vi "GPS.vi"() -> (0 "GPS error out":errorcluster caption="error out")   [LabVIEW 2016]
uses:
  DLL/Checksum_(T_F).dll
panel:
  in  "stop?":bool
  in  "GPS error in":errorcluster
  in  "GPS Baud rate":u32(ring)=38400 items=["Auto Connect"=0, "300"=300, "600"=600, "1200"=1200, "2400"=2400, "4800"=4800, "9600"=9600, "19200"=19200, "38400"=38400, "57600"=57600, "115200"=115200]
  out "GPS port out":refnum<visa-resource-name>
  out "Time":string
  out "N/S":string
  out "E/W":string
  out "Chechsum 부분":string
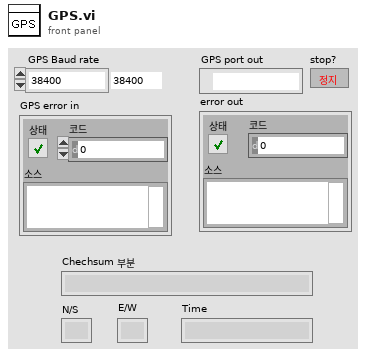
[diagram p1: front panel]
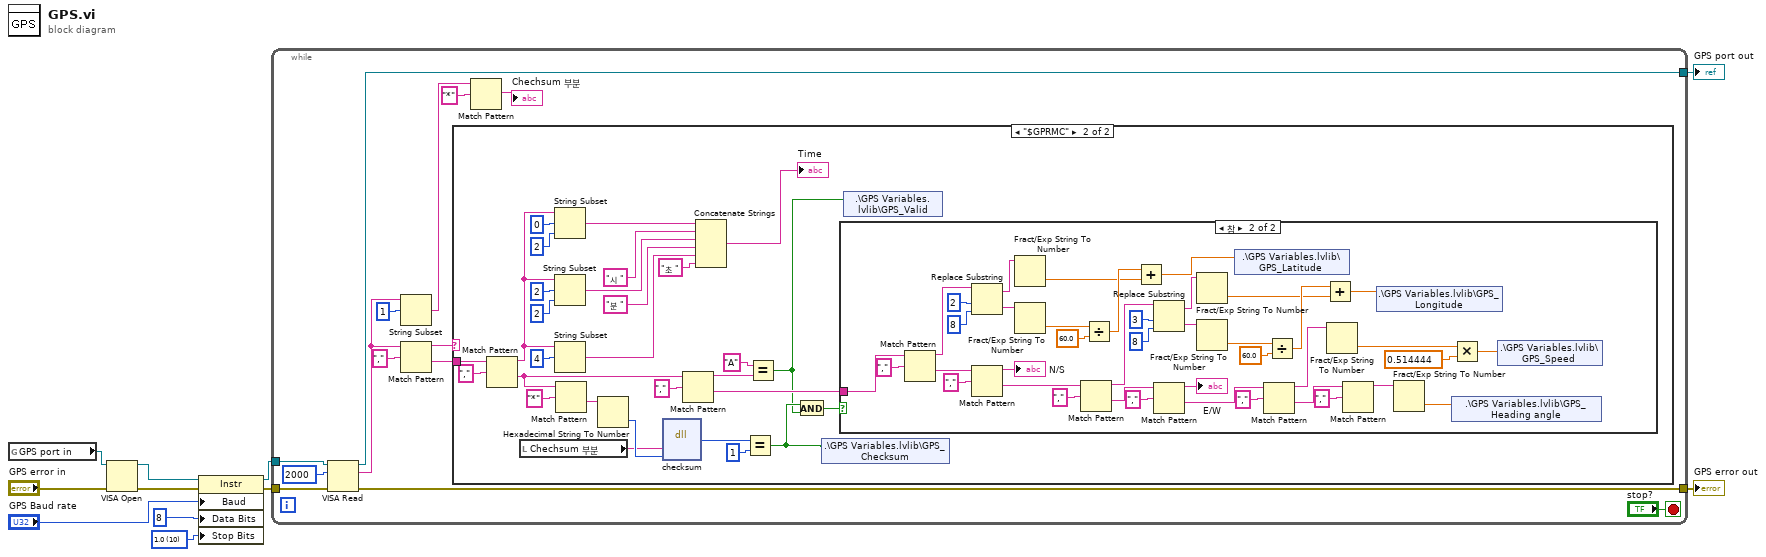
[diagram p0: block diagram]
diagram:
  w8 = u16 10 items=["1.0"=10, "1.5"=15, "2.0"=20] ("Serial Settings:Stop Bits")
  n1 = global read "[GV]_GPS Port NUM.vi" "GPS port in"() -> (w1:refnum<visa-resource-name>)
  n2 = VISA Open(error in (no error)="GPS error in", VISA resource name=w1) -> (VISA resource name=w2:refnum<visa-resource-name>, error out=w6:errorcluster)  [unwired: 3 in]
  n3 = property class="Instr"(reference=w2, error in=w6, "Baud"="GPS Baud rate", "Data Bits"=u16 8 ("Serial Settings:Data Bits"), "Stop Bits"=w8) -> (reference out=w4:refnum<visa-resource-name>, error out=w3:errorcluster)
  n4 = while {
    tunnel: w4 -> [w17]
    tunnel: w3 -> [w16]
    tunnel: [w14] -> w10
    tunnel: [w13] -> w11
    stop <- "stop?" stop-if-true
    n5 = VISA Read(VISA resource name=w17, byte count=u32 2000 ("바이트 카운트"), error in (no error)=w16) -> (VISA resource name out=w14:refnum<visa-resource-name>, read buffer=w18:string, error out=w13:errorcluster)  [unwired: 1 out]
    n6 = String Subset(string=w18, offset (0)=1 ("오프셋(0)")) -> (substring=w19:string)  [unwired: 1 in]
    n7 = Match Pattern(string=w18, regular expression="," ("정규식")) -> (before substring=w24:string, after substring=w23:string)  [unwired: 1 in, 2 out]
    n8 = case shown="\"$GPRMC\"" w24 {
      tunnel: w23 -> [_ w53]
      frame "거짓", Default {
      }
      frame "$GPRMC" {
        n9 = Match Pattern(string=w53, regular expression="," ("정규식")) -> (before substring=w38:string, after substring=w35:string)  [unwired: 1 in, 2 out]
        n10 = local read "Chechsum 부분"() -> (w28:string)
        n11 = String Subset(string=w38, offset (0)=0 ("오프셋(0)"), length (rest)=2 ("길이(나머지)")) -> (substring=w44:string)
        n12 = String Subset(string=w38, offset (0)=2 ("오프셋(0)"), length (rest)=2 ("길이(나머지)")) -> (substring=w47:string)
        n13 = String Subset(string=w38, offset (0)=4 ("오프셋(0)")) -> (substring=w50:string)  [unwired: 1 in]
        n14 = Match Pattern(string=w35, regular expression="*" ("정규식")) -> (after substring=w31:string)  [unwired: 1 in, 3 out]
        n15 = Hexadecimal String To Number(string=w31) -> (number=w34:u32)  [unwired: 2 in, 1 out]
        n16 = dll-call lib="PTH2abs CUsersuserDesktop[Github]_GPS Teamlabview_program(ììì¤ì¸ ëª¨ë  Vi, dllíì¼ ëª¨ìì ì²´íë¡ê·¸ë¨DLLChecksum_(T_F).dll" fn="checksum"("NMEA string"=w28, "Checksum"=w34) -> ("반환 타입"=w33:i16)  [unwired: 5 in, 2 out]
        n17 = Match Pattern(string=w35, regular expression="," ("정규식")) -> (before substring=w37:string, after substring=w29:string)  [unwired: 1 in, 2 out]
        n18 = Concatenate Strings(w44, "시 ", w47, "분 ", w50, "초 ") -> (→"Time":string)
        n19 = Equal?(x=w33, y=i16 1) -> (x = y?=w27:bool)
        n20 = Equal?(x="A" ("y"), y=w37) -> (x = y?=w26:bool)
        n21 = And(x=w27, y=w26) -> (x .and. y?=w30:bool)
        n22 = shared-variable ".\\GPS Variables.lvlib\\GPS_Checksum"(w27) -> ()  [unwired: 1 in, 1 out]
        n23 = case shown="참" w30 {
          tunnel: w29 -> [_ w94]
          frame False {
          }
          frame True {
            n24 = Match Pattern(string=w94, regular expression="," ("정규식")) -> (before substring=w76:string, after substring=w75:string)  [unwired: 1 in, 2 out]
            n25 = Replace Substring(2:8 ("위도_길이(부분 문자열의 길이)"), 3:2 ("위도_오프셋"), 5:w76) -> (0:w88:string, 1:w87:string)  [unwired: 1 in]
            n26 = Match Pattern(string=w75, regular expression="," ("정규식")) -> (before substring=→"N/S":string, after substring=w72:string)  [unwired: 1 in, 2 out]
            n27 = Fract/Exp String To Number(string=w87) -> (number=w85:dbl)  [unwired: 1 in, 3 out]
            n28 = Fract/Exp String To Number(string=w88) -> (number=w89:dbl)  [unwired: 1 in, 3 out]
            n29 = Match Pattern(string=w72, regular expression="," ("정규식")) -> (before substring=w71:string, after substring=w68:string)  [unwired: 1 in, 2 out]
            n30 = Divide(x=w89, y=60.0) -> (x/y=w86:dbl)
            n31 = Add(x=w86, y=w85) -> (x+y=w57:dbl)
            n32 = Replace Substring(2:8 ("경도_길이(부분 문자열의 길이)"), 3:3 ("경도_오프셋(0)"), 5:w71) -> (0:w81:string, 1:w80:string)  [unwired: 1 in]
            n33 = Match Pattern(string=w68, regular expression="," ("정규식")) -> (before substring=→"E/W":string, after substring=w65:string)  [unwired: 1 in, 2 out]
            n34 = Fract/Exp String To Number(string=w80) -> (number=w78:dbl)  [unwired: 4 out]
            n35 = Fract/Exp String To Number(string=w81) -> (number=w70:dbl)  [unwired: 4 out]
            n36 = shared-variable ".\\GPS Variables.lvlib\\GPS_Latitude"(w57) -> ()  [unwired: 1 in, 1 out]
            n37 = Match Pattern(string=w65, regular expression="," ("정규식")) -> (before substring=w62:string, after substring=w60:string)  [unwired: 1 in, 2 out]
            n38 = Divide(x=w70, y=60.0) -> (x/y=w79:dbl)
            n39 = Add(x=w79, y=w78) -> (x+y=w56:dbl)
            n40 = Fract/Exp String To Number(string=w62) -> (number=w63:dbl)  [unwired: 3 in, 1 out]
            n41 = Match Pattern(string=w60, regular expression="," ("정규식")) -> (before substring=w59:string)  [unwired: 1 in, 3 out]
            n42 = shared-variable ".\\GPS Variables.lvlib\\GPS_Longitude"(w56) -> ()  [unwired: 1 in, 1 out]
            n43 = Fract/Exp String To Number(string=w59) -> (number=w58:dbl)  [unwired: 3 in, 1 out]
            n44 = Multiply(x=w63, y=0.514444) -> (x*y=w55:dbl)
            n45 = shared-variable ".\\GPS Variables.lvlib\\GPS_Heading angle"(w58) -> ()  [unwired: 1 in, 1 out]
            n46 = shared-variable ".\\GPS Variables.lvlib\\GPS_Speed"(w55) -> ()  [unwired: 1 in, 1 out]
          }
        }
        n47 = shared-variable ".\\GPS Variables.lvlib\\GPS_Valid"(w26) -> ()  [unwired: 1 in, 1 out]
      }
    }
    n48 = Match Pattern(string=w19, regular expression="*" ("정규식")) -> (before substring=→"Chechsum 부분":string)  [unwired: 1 in, 3 out]
  }
  "GPS error out" <- w11
  "GPS port out" <- w10
